vi "ru_duilie.vi"(6 "yw":string, 7 "name":string, 8 "sp_shuoming":string, 9 "sp_yijian":string, 10 "id":string, 11 "lc_num":string) -> (1 "error":errorcluster={"status"=TRUE, "code"=255, "source"="非法操作！"})   [LabVIEW 2017, in "Lib_code.lvlib"]
uses:
  Lib_code.lvlib
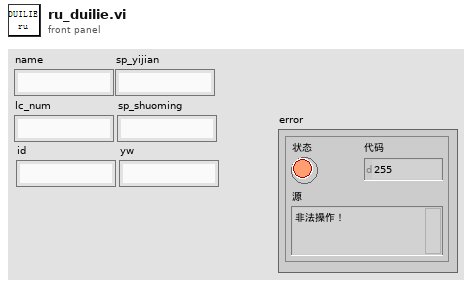
[diagram p1: front panel]
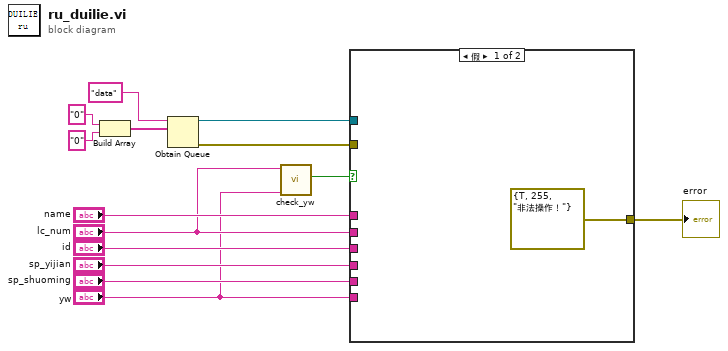
[diagram p0: block diagram]
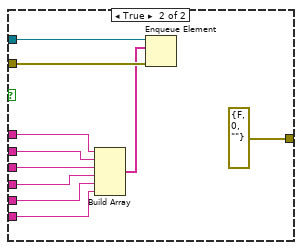
[diagram p2: hidden frame]
diagram:
  n1 = Build Array("0" ("元素"), "0" ("元素")) -> (w11:string[])
  n2 = Obtain Queue(name (unnamed)="data" ("名称（未命名）"), element data type=w11) -> (queue out=w10:refnum<queue>, error out=w9:errorcluster)  [unwired: 3 in, 1 out]
  n3 = call "check_yw.vi"("yw"="yw", "lc_num"="lc_num") -> ("check_yw"=w2:bool)  [unwired: 8 in, 1 out]
  n4 = case shown="假" w2 {
    tunnel: w10 -> [_ w25]
    tunnel: w9 -> [_ w24]
    tunnel: "name" -> [_ w22]
    tunnel: "id" -> [_ w21]
    tunnel: "sp_yijian" -> [_ w20]
    tunnel: "sp_shuoming" -> [_ w19]
    tunnel: "lc_num" -> [_ w18]
    tunnel: "yw" -> [_ w17]
    tunnel: [errorcluster {"status"=TRUE, "code"=255, "source"="非法操作！"} ("error 3") errorcluster {"status"=FALSE, "code"=0, "source"=""} ("error")] -> w1
    frame False {
    }
    frame True {
      n5 = Build Array(w22, w18, w21, w20, w19, w17) -> (w23:string[])
      n6 = Enqueue Element(queue=w25, element=w23, error in (no error)=w24) -> ()  [unwired: 1 in, 3 out]
    }
  }
  "error" <- w1
